vi "goToStandby.vi"(8 "error in (no error)":errorcluster, 10 "model":refnum<class "Model.lvclass">, 11 "EnabledState in":refnum<class "EnabledState.lvclass">) -> (0 "error out":errorcluster, 2 "model 2":refnum<class "Model.lvclass">, 3 "EnabledState out":refnum<class "EnabledState.lvclass">)   [LabVIEW 2013, in "EnabledState.lvclass"]
uses:
  EnabledState.lvclass
  Model/Model/Model.lvclass
  Typedefs/StateSelector.ctl
  Typedefs/M2AADTTypedefs.lvlib
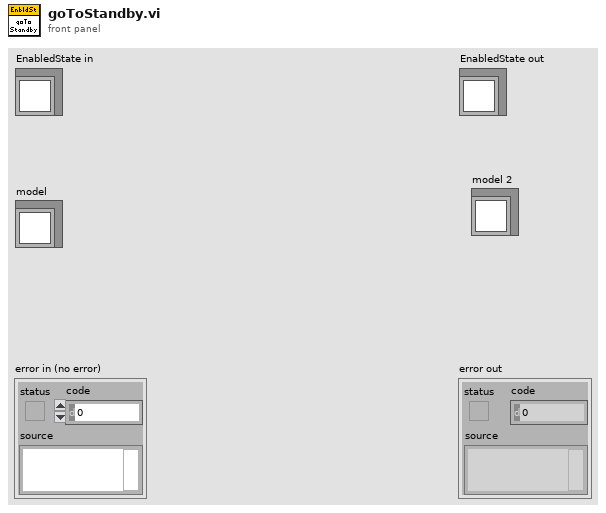
[diagram p1: front panel]
types:
  T1 = typedef "M2AADTTypedefs.lvlib/StateSelector.ctl" = enum16{"EndingCycleState", "FaultState", "InteractiveMotionState", "MovingToNewForceState", "OffState", "PausingState", "StandbyState", "StoppedState"}
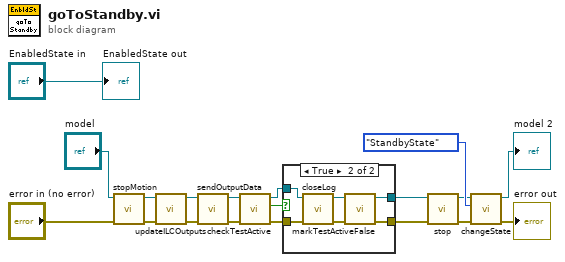
[diagram p0: block diagram]
diagram:
  n1 = call "stopMotion.vi"("error in (no error)"="error in (no error)", "Model in"="model") -> ("error out"=w8:errorcluster, "Model out"=w10:refnum<class "Model.lvclass">)  [unwired: 8 in]
  n2 = call "updateILCOutputs.vi"("error in (no error)"=w8, "Model in"=w10) -> ("error out"=w7:errorcluster, "Model out"=w9:refnum<class "Model.lvclass">)  [unwired: 8 in]
  n3 = call "sendOutputData.vi"("error in (no error)"=w7, "Model in"=w9) -> ("error out"=w5:errorcluster, "Model out"=w6:refnum<class "Model.lvclass">)  [unwired: 8 in]
  n4 = call "checkTestActive.vi"("error in (no error)"=w5, "Model in"=w6) -> ("error out"=w11:errorcluster, "testActiveIsTrue"=w13:bool, "Model out"=w12:refnum<class "Model.lvclass">)  [unwired: 7 in]
  n5 = case shown="True" w13 {
    tunnel: [w21 w24] -> w4
    tunnel: [w20 w22] -> w2
    tunnel: w12 -> [w21 w27]
    tunnel: w11 -> [w20 w26]
    frame False {
    }
    frame True {
      n6 = call "closeLog.vi"("error in (no error)"=w26, "Model in"=w27) -> ("error out"=w23:errorcluster, "Model out"=w25:refnum<class "Model.lvclass">)  [unwired: 8 in]
      n7 = call "markTestActiveFalse.vi"("error in (no error)"=w23, "Model in"=w25) -> ("error out"=w22:errorcluster, "Model out"=w24:refnum<class "Model.lvclass">)  [unwired: 8 in]
    }
  }
  n8 = call "stop.vi"("error in (no error)"=w2, "Model in"=w4) -> ("error out"=w1:errorcluster, "Model out"=w3:refnum<class "Model.lvclass">)  [unwired: 8 in]
  n9 = call "changeState.vi"("error in (no error)"=w1, "State:"=StateSelector."StandbyState", "Model in"=w3) -> ("error out"=→"error out":errorcluster, "Model out"=→"model 2":refnum<class "Model.lvclass">)  [unwired: 7 in]
  "EnabledState out" <- "EnabledState in"
